vi "Pre Launch Init.vi"(11 "Nested in":refnum<class "DisplayerUI.lvclass">) -> (0 "error out":errorcluster, 3 "Nested out":refnum<class "DisplayerUI.lvclass">)   [LabVIEW 2020, in "Displayer.lvlib" / "DisplayerUI.lvlib" / "DisplayerUI.lvclass"]
doc: "(<B>Filename</B>: Actor Framework.lvlib:Actor.lvclass:Pre Launch Init.vi)\n\nDefines behavior that occurs after the Launch Nested Actor method is invoked but before the actor's Actor Core method begins running.\n\nBy default, this method does nothing. A descendant class may override it to define behavior."
uses:
  DisplayerUI.lvclass
  DisplayerUI.lvclass/DisplayerUI.ctl
  <vilib>/ActorFramework/Actor/Actor.lvclass
  <vilib>/vision/Image Controls.llb/IMAQ Image.ctl
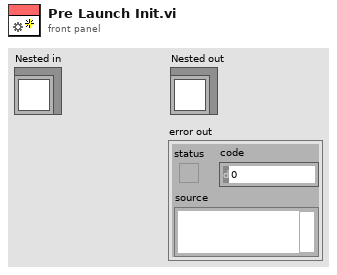
[diagram p1: front panel]
types:
  T1 = typedef "IMAQ Image.ctl" = refnum<image>
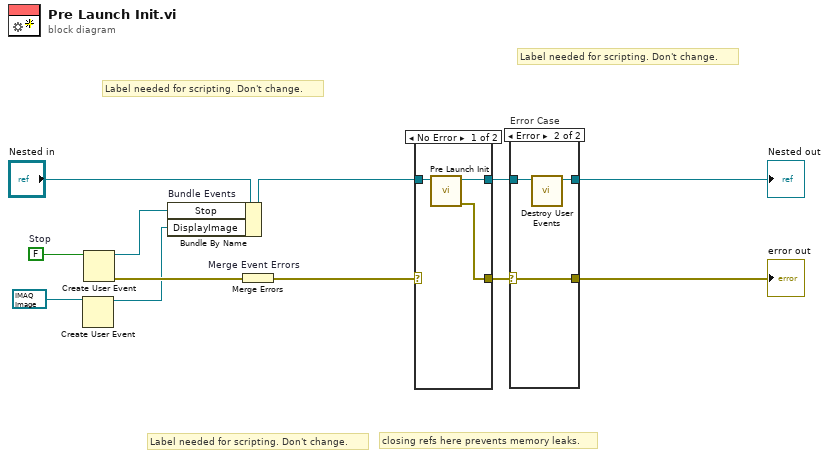
[diagram p0: block diagram]
diagram:
  w11 = FALSE  # Stop
  # "Label needed for scripting. Don't change."
  # "Label needed for scripting. Don't change."
  # "Label needed for scripting. Don't change."
  # "closing refs here prevents memory leaks."
  n1 = Create User Event(user event datatype=T1 refnum ("RawImage")) -> (user event=w1:refnum<user-event>)  [unwired: 1 in, 1 out]
  n2 = Create User Event(user event datatype=w11) -> (user event=w8:refnum<user-event>, error out=w10:errorcluster)  [unwired: 1 in]
  n3 = Bundle By Name "Bundle Events"(cluster="Nested in", "Stop"=w8, "DisplayImage"=w1) -> (w5:refnum<class "DisplayerUI.lvclass">)
  n4 = Merge Errors "Merge Event Errors"(w10) -> (w4:errorcluster)
  n5 = case shown="No Error" w4 {
    selector: w4 -> [_ w17]
    tunnel: [w15 w16] -> w6
    tunnel: w5 -> [w14 w16]
    tunnel: [w13 w17] -> w3
    frame No Error {
      n6 = call-parent "Pre Launch Init.vi"("Actor in"=w14) -> ("error out"=w13:errorcluster, "Actor out"=w15:refnum<class "DisplayerUI.lvclass">)  [unwired: 9 in]
    }
    frame Error {
    }
  }
  n7 = case "Error Case" shown="Error" w3 {
    selector: w3 -> [w18 w22]
    tunnel: w6 -> [w19 w21]
    tunnel: [w19 w20] -> w9
    tunnel: [w18 w22] -> w7
    frame No Error {
    }
    frame Error {
      n8 = call "Destroy User Events.vi"("UI Template in"=w21) -> ("UI Template out"=w20:refnum<class "DisplayerUI.lvclass">)  [unwired: 10 in]
    }
  }
  "error out" <- w7
  "Nested out" <- w9
